vi "表格显示内容刷新V2.vi"(8 "数据模式":bool, 9 "表格":string[][](table), 10 "CANBURF":u32[][](array[numeric]), 11 "当前显示表格总行数":i32) -> (3 "输出数组":string[][](array[string]))   [LabVIEW 2021]
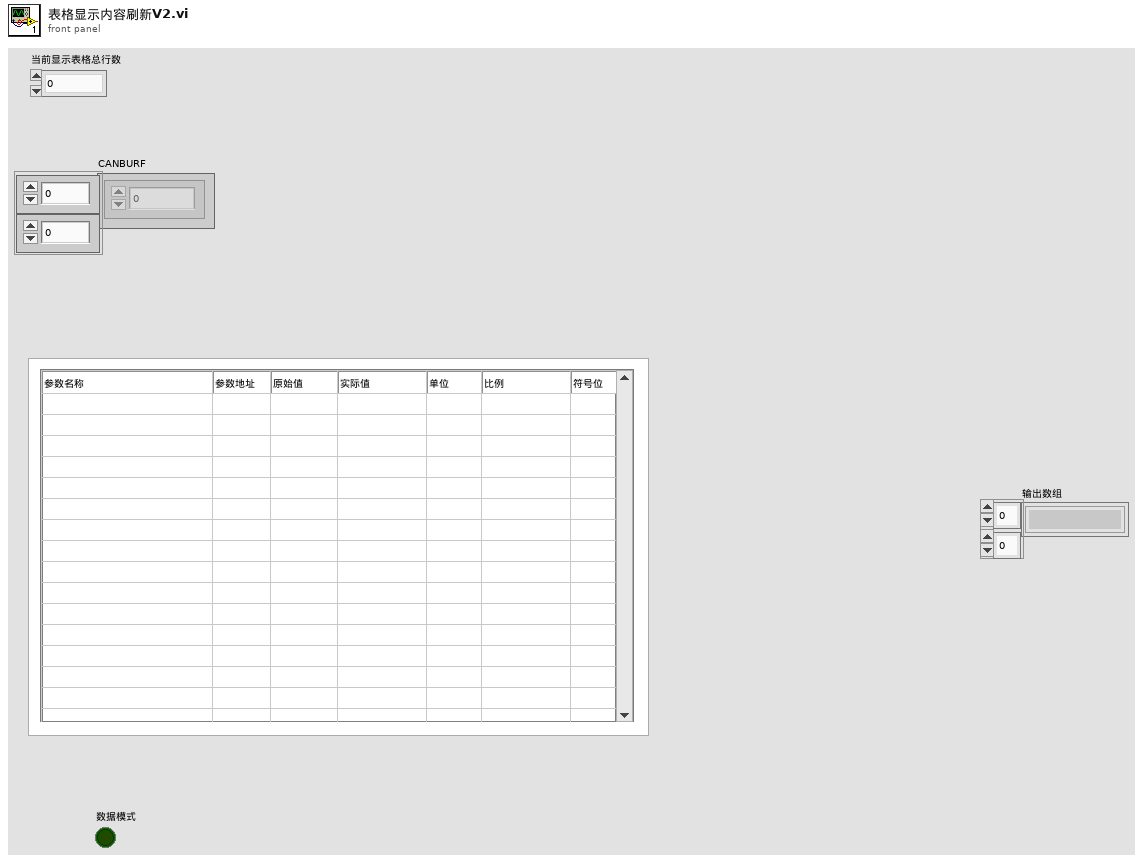
[diagram p1: front panel]
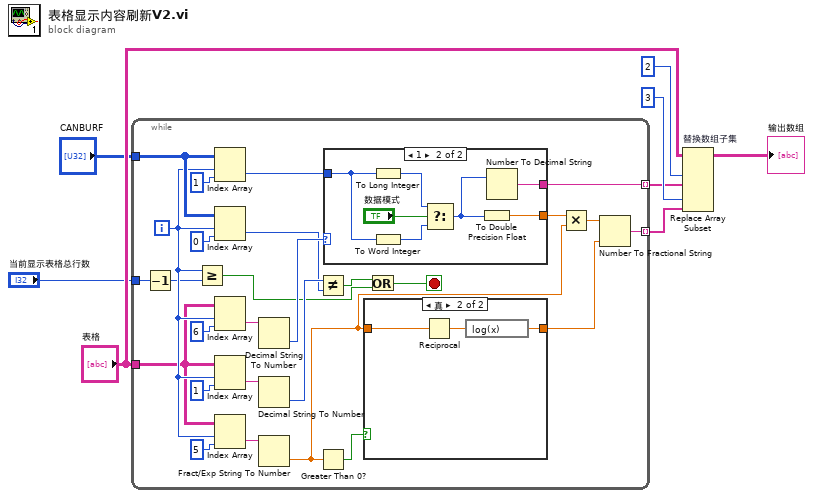
[diagram p0: block diagram]
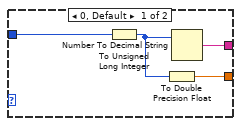
[diagram p2: hidden frame]
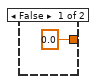
[diagram p3: hidden frame]
diagram:
  n1 = while {
    tunnel: "CANBURF" -> [w24]
    tunnel: [w13] -> w6 mode=indexing
    tunnel: [w12] -> w5 mode=indexing
    tunnel: "表格" -> [w10]
    tunnel: "当前显示表格总行数" -> [w9]
    i -> [w21]
    stop <- w14 stop-if-true
    n2 = Decrement(x=w9) -> (x-1=w11:i32)
    n3 = Greater Or Equal?(x=w21, y=w11) -> (x >= y?=w15:bool)
    n4 = Index Array(array=w24, index (row)=w21, index (col)=1 ("禁用的索引 (列)")) -> (element=w33:u32)
    n5 = Index Array(array=w24, index (row)=w21, index (col)=0 ("禁用的索引 (列)")) -> (element=w17:u32)
    n6 = Index Array(array=w10, index (row)=w21, index (col)=6 ("索引")) -> (element=w27:string)
    n7 = Index Array(array=w10, index (row)=w21, index (col)=1 ("禁用的索引 (列)")) -> (element=w19:string)
    n8 = Index Array(array=w10, index (row)=w21, index (col)=5 ("索引")) -> (element=w32:string)
    n9 = Decimal String To Number(string=w27) -> (number=w25:i32)  [unwired: 2 in, 1 out]
    n10 = Decimal String To Number(string=w19) -> (number=w18:i32)  [unwired: 2 in, 1 out]
    n11 = Fract/Exp String To Number(string=w32) -> (number=w28:dbl)  [unwired: 3 in, 1 out]
    n12 = Not Equal?(x=w18, y=w17) -> (x != y?=w16:bool)
    n13 = Greater Than 0?(x=w28) -> (x > 0?=w30:bool)
    n14 = case shown="1" w25 {
      tunnel: w33 -> [w39 w42]
      tunnel: [w37 w46] -> w26
      tunnel: [w36 w45] -> w13
      frame 0, Default {
        n15 = To Unsigned Long Integer(number=w39) -> (unsigned 32bit integer=w38:u32)
        n16 = To Double Precision Float(number=w38) -> (double precision float=w37:dbl)
        n17 = Number To Decimal String(number=w38) -> (decimal integer string=w36:string)  [unwired: 1 in]
      }
      frame 1 {
        n18 = To Long Integer(number=w42) -> (32bit integer=w43:i32)
        n19 = To Word Integer(number=w42) -> (16bit integer=w41:i16)
        n20 = Select(t=w43, s="数据模式", f=w41) -> (s? t:f=w44:i32)
        n21 = To Double Precision Float(number=w44) -> (double precision float=w46:dbl)
        n22 = Number To Decimal String(number=w44) -> (decimal integer string=w45:string)  [unwired: 1 in]
      }
    }
    n23 = case shown="真" w30 {
      tunnel: w28 -> [_ w50]
      tunnel: [0.0 w48] -> w29
      frame False {
      }
      frame True {
        n24 = Reciprocal(x=w50) -> (1/x=w49:dbl)
        n25 = expression code="log(x)"(w49) -> (w48:dbl)
      }
    }
    n26 = Or(x=w16, y=w15) -> (x .or. y?=w14:bool)
    n27 = Multiply(x=w26, y=w28) -> (x*y=w31:dbl)
    n28 = Number To Fractional String(number=w31, precision (6)=w29) -> (F-format string=w12:string)  [unwired: 2 in]
  }
  n29 = Replace Array Subset "替换数组子集"(array="表格", new element #1=w6, index (col) #1=2 ("禁用的索引 (列)"), new element #2=w5, index (col) #2=3 ("索引 (列)")) -> (→"输出数组":string[][])  [unwired: 2 in]
